vi "COMMAND_Status.vi"(8 "error in (no error)":errorcluster, 11 "StageDL090602SutterMP285 in":refnum<class "StageMMS2015ASI.lvclass">) -> (0 "error out":errorcluster, 2 "status":T1, 3 "StageDL090602SutterMP285 out":refnum<class "StageMMS2015ASI.lvclass">)   [LabVIEW 2010, in "StageMMS2015ASI.lvclass"]
uses:
  StageMMS2015ASI.lvclass
  status_cluster.ctl
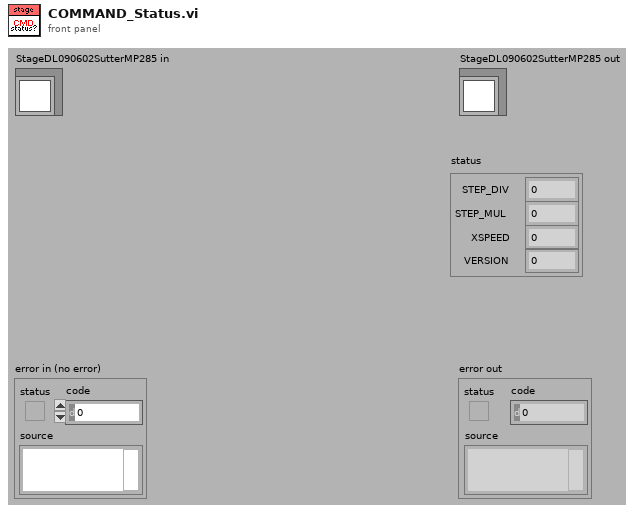
[diagram p1: front panel]
types:
  T1 = typedef "StageMMS2015ASI.lvclass/status_cluster.ctl" = cluster{"STEP_DIV":i32, "STEP_MUL":i32, "XSPEED":i32, "VERSION":i32}
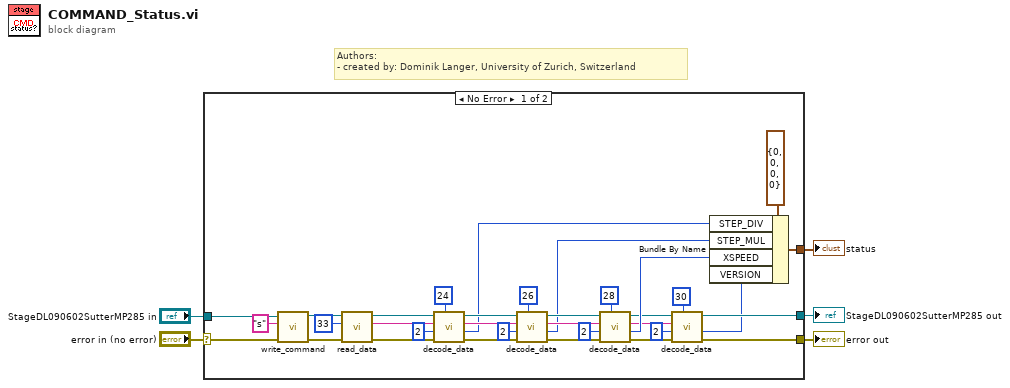
[diagram p0: block diagram]
diagram:
  # "Authors: \n- created by: Dominik Langer, University of Zurich, Switzerland"
  n1 = case shown="No Error" "error in (no error)" {
    selector: "error in (no error)" -> [w35 w41]
    tunnel: [w12 w41] -> w4
    tunnel: [w10 w40] -> w2
    tunnel: "StageDL090602SutterMP285 in" -> [w34 w40]
    tunnel: [w15 _] -> w1
    frame No Error {
      n2 = call-dynamic "write_command.vi"("error in (no error)"=w35, "command (without terminating \"\\n\")"="s" ("command (without terminating \"\\n\")"), "DL090602SutterMP285Stage in"=w34) -> ("error out"=w36:errorcluster, "DL090602SutterMP285Stage out"=w38:refnum<class "StageMMS2015ASI.lvclass">)  [unwired: 7 in]
      n3 = call-dynamic "read_data.vi"("error in (no error)"=w36, "bytes to read"=u32 33, "DL090602SutterMP285Stage in"=w38) -> ("error out"=w33:errorcluster, "hex data string"=w6:string, "DL090602SutterMP285Stage out"=w32:refnum<class "StageMMS2015ASI.lvclass">)  [unwired: 6 in]
      n4 = call-dynamic "decode_data.vi"("offset"=24, "error in (no error)"=w33, "length"=2, "encoded data string in"=w6, "DL090602SutterMP285Stage in"=w32) -> ("error out"=w26:errorcluster, "decoded data"=w18:i32, "encoded data string out"=w21:string, "DL090602SutterMP285Stage out"=w20:refnum<class "StageMMS2015ASI.lvclass">)  [unwired: 3 in]
      n5 = call-dynamic "decode_data.vi"("offset"=26, "error in (no error)"=w26, "length"=2, "encoded data string in"=w21, "DL090602SutterMP285Stage in"=w20) -> ("error out"=w27:errorcluster, "decoded data"=w17:i32, "encoded data string out"=w22:string, "DL090602SutterMP285Stage out"=w24:refnum<class "StageMMS2015ASI.lvclass">)  [unwired: 3 in]
      n6 = call-dynamic "decode_data.vi"("offset"=28, "error in (no error)"=w27, "length"=2, "encoded data string in"=w22, "DL090602SutterMP285Stage in"=w24) -> ("error out"=w13:errorcluster, "decoded data"=w16:i32, "encoded data string out"=w9:string, "DL090602SutterMP285Stage out"=w11:refnum<class "StageMMS2015ASI.lvclass">)  [unwired: 3 in]
      n7 = call-dynamic "decode_data.vi"("offset"=30, "error in (no error)"=w13, "length"=2, "encoded data string in"=w9, "DL090602SutterMP285Stage in"=w11) -> ("error out"=w12:errorcluster, "decoded data"=w7:i32, "DL090602SutterMP285Stage out"=w10:refnum<class "StageMMS2015ASI.lvclass">)  [unwired: 3 in, 1 out]
      n8 = Bundle By Name(cluster=T1 {"STEP_DIV"=0, "STEP_MUL"=0, "XSPEED"=0, "VERSION"=0} ("status"), "STEP_DIV"=w18, "STEP_MUL"=w17, "XSPEED"=w16, "VERSION"=w7) -> (w15:T1)
    }
    frame Error {
    }
  }
  "error out" <- w4
  "StageDL090602SutterMP285 out" <- w2
  "status" <- w1
